vi "Test RedCase_FlashUpdate_Run.bat.vi"(8 "error in (no error)":errorcluster, 9 "SN":string="ABCSN", 10 "RedCase Auto Path":string=".\\RedCase_Auto\\Debug\\FlashUpdate_Run.bat", 11 "Bin":string=".\\RedCase_Auto\\Debug\\HX6330B03_C_Sharp_GM_Mobis_2992x1299_16.3_Falcon_20251223_S1C7A404_Test_Ver4-0.bin") -> (0 "error out":errorcluster, 2 "RecCase Log Path":string, 3 "Result":bool)   [LabVIEW 2024]
uses:
  <vilib>/Utility/error.llb/Trim Whitespace One-Sided.vi
panel:
  out "output Str":string="@echo off\nsetlocal enabledelayedexpansion\n\nREM ========= 用户可配置区 =========\nset RFP_DIR=C:\\Program Files (x86)\\Renesas Electronics\\Programming Tools\\Renesas Flash Programmer V3.16\nset RFP_EXE=%RFP_DIR%\\RFPV3.exe\nset RFP_CONSOLE=%RFP_DIR%\\RFPV3.Console.exe\n\nset PROJECT=D:\\Alvin\\1.Project\\5.ZhiRuiJia\\Flash\\RFP_Auto\\Project\\k7001.rpj\nREM 固件已配置在 .rpj 内，这里默认不再单独指定 /file\nset FIRMWARE=\nset LOG_DIR=D:\\Alvin\\1.Project\\5.ZhiRuiJia\\Flash\\RFP_Auto\\Logs\nset RETRY=2\nREM 可选：如果你只有一台E2 Lite，通常不需要指定tool序列号\nset TOOL_SN=\nREM 示例：set TOOL_SN=xxxxxxxxx\nREM =================================\n\nif not exist \"%LOG_DIR%\" mkdir \"%LOG_DIR%\"\n\nREM SN 可由扫码枪/上位机传入：flash_once.bat SNABCSN\nset SN=%1\nif \"%SN%\"==\"\" set SN=NO_SN\n\nREM 时间戳（yyyyMMdd_HHmmss）\nfor /f %%i in ('powershell -NoProfile -Command \"Get-Date -Format yyyyMMdd_HHmmss\"') do set TS=%%i\n\nset LOG_FILE=%LOG_DIR%\\%SN%_%TS%.log\n\necho [INFO] SN=%SN%\necho [INFO] Project=%PROJECT%\nif not \"%FIRMWARE%\"==\"\" echo [INFO] Firmware=%FIRMWARE%\necho [INFO] Log=%LOG_FILE%\necho.\n\nREM 参数拼接\nset COMMON_ARGS=/silent \"%PROJECT%\" /command epv /log \"%LOG_FILE%\"\nif not \"%FIRMWARE%\"==\"\" set COMMON_ARGS=%COMMON_ARGS% /file \"%FIRMWARE%\"\nif not \"%TOOL_SN%\"==\"\" set COMMON_ARGS=%COMMON_ARGS% /tool %TOOL_SN%\n\nset /a COUNT=0\n\n:RETRY_LOOP\nset /a COUNT+=1\necho [INFO] Attempt !COUNT! ...\n\nREM 优先用 RFPV3.exe /silent\n\"%RFP_EXE%\" %COMMON_ARGS%\nset RC=%ERRORLEVEL%\n\necho [INFO] ExitCode=%RC%\n\nif \"%RC%\"==\"0\" goto PASS\n\nif !COUNT! LEQ %RETRY% (\n    echo [WARN] Programming failed, retrying...\n    timeout /t 2 >nul\n    goto RETRY_LOOP\n)\n\ngoto FAIL\n\n:PASS\nfor /f %%i in ('powershell -NoProfile -Command \"Get-Date -Format yyyyMMdd_HHmmss\"') do set END_TS=%%i\necho [INFO] EndTime=%END_TS%\necho [PASS] %SN% %TS% >> \"%LOG_DIR%\\summary_pass.txt\"\necho SUCCESS\nexit /b 0\n\n:FAIL\nfor /f %%i in ('powershell -NoProfile -Command \"Get-Date -Format yyyyMMdd_HHmmss\"') do set END_TS=%%i\necho [INFO] EndTime=%END_TS%\necho [FAIL] %SN% %TS% ExitCode=%RC% >> \"%LOG_DIR%\\summary_fail.txt\"\necho FAIL\nexit /b 1\r\n"
  out "path":path=path "D:/WeiFu/Labview ATS/Customer_Zhuo/RF_Download/ATS/Project/RFP_Auto/Scripts/Flash_once.bat"
  out "result string":string
  # "D:\\WeiFu\\Labview ATS\\Customer_Zhuo\\RF_Download\\ATS\\Project\\RFP_Auto\\Scripts\\Flash_once.bat"
  # "..\\RFP_Auto\\Scripts\\Flash_once.bat"
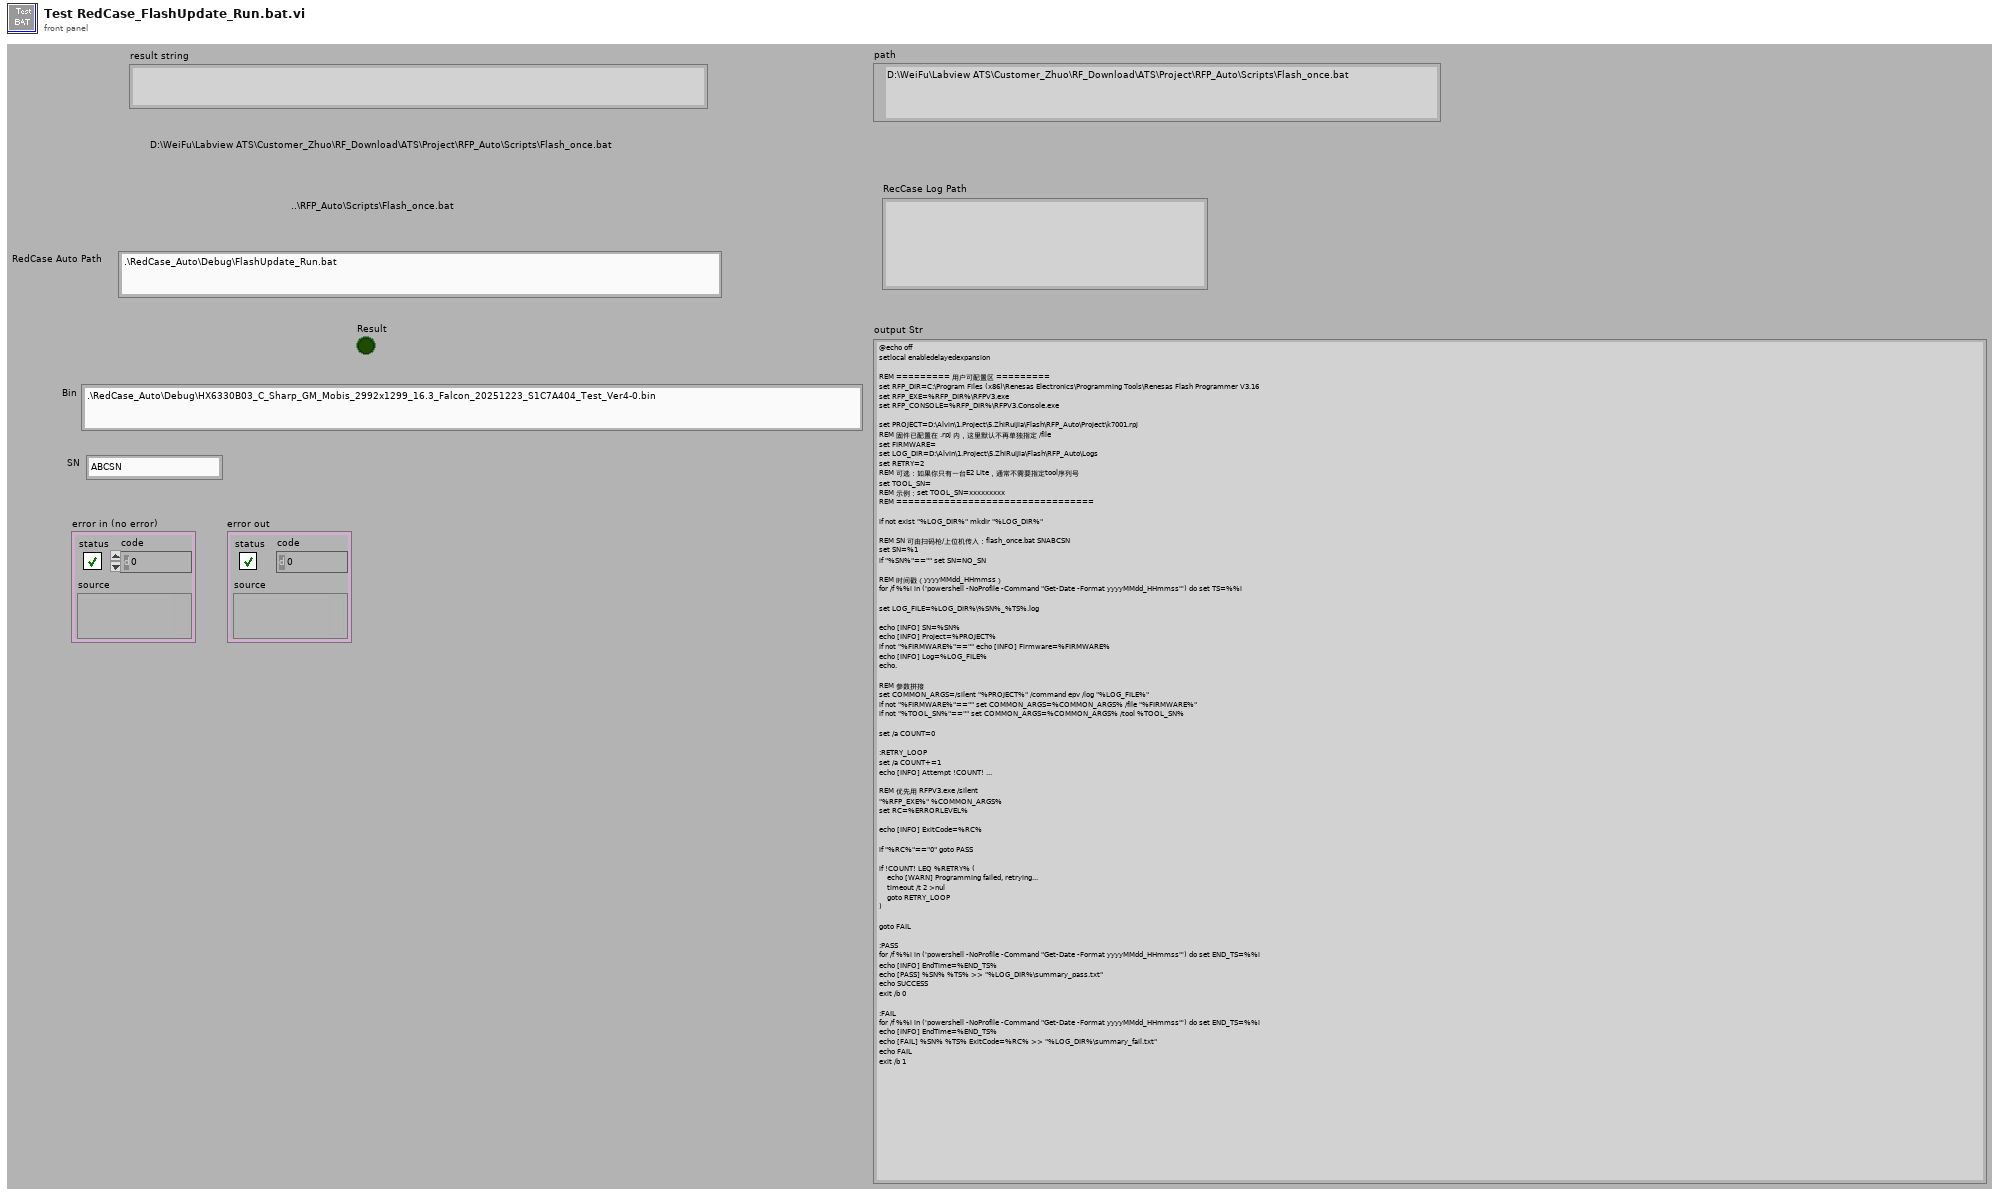
[diagram p1: front panel]
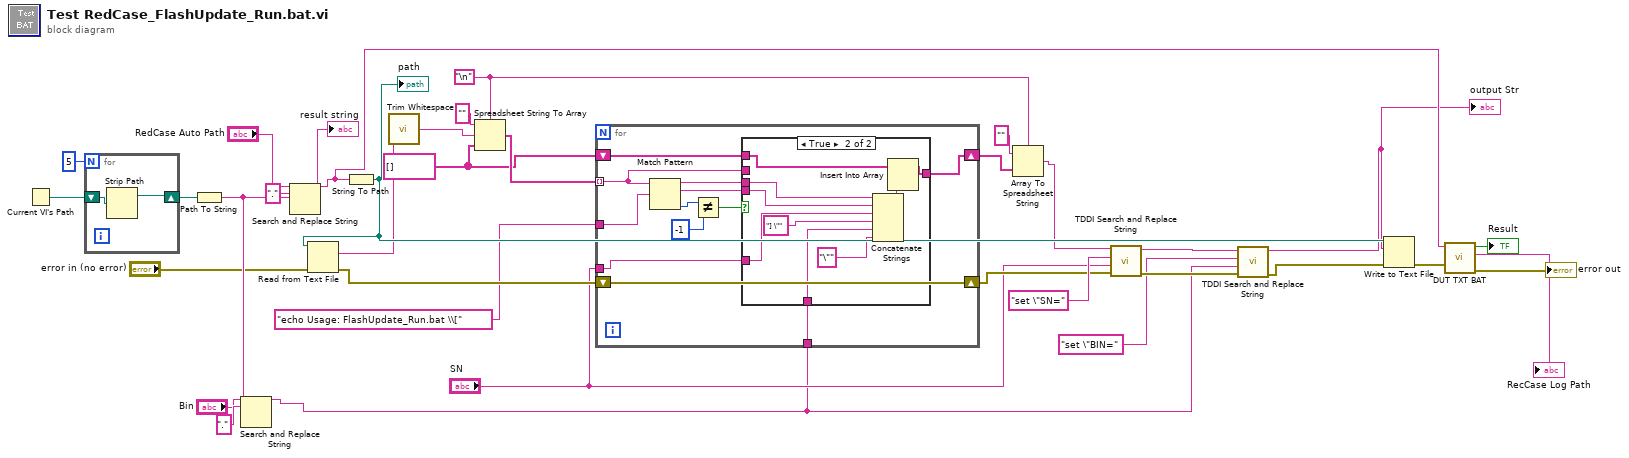
[diagram p0: block diagram]
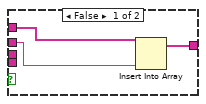
[diagram p2: hidden frame]
diagram:
  w18 = string[] []
  w15 = "\n"
  n1 = Current VI's Path() -> (path=w33:path)
  n2 = for {
    N: 5 -> [_]
    shift-right: [w36] -> w31
    shift-left: w33 -> [w37]
    n3 = Strip Path(path=w37) -> (stripped path=w36:path)  [unwired: 1 out]
  }
  n4 = Path To String(path=w31) -> (string=w26:string)
  n5 = Search and Replace String(input string="Bin", search string=".", replace string=w26) -> (result string=w1:string)  [unwired: 5 in, 3 out]
  n6 = Search and Replace String(input string="RedCase Auto Path", search string=".", replace string=w26) -> (result string=w11:string)  [unwired: 5 in, 3 out]
  "result string" <- w11
  n7 = String To Path(string=w11) -> (path=w22:path)
  "path" <- w22
  n8 = Read from Text File(file (use dialog)=w22, error in="error in (no error)") -> (text=w14:string, error out=w13:errorcluster)  [unwired: 2 in, 2 out]
  n9 = call <vilib>:"Trim Whitespace.vi"("string"=w14) -> ("trimmed string"=w20:string)  [unwired: 1 in]
  n10 = Spreadsheet String To Array(delimiter (Tab)=w15, format string="", spreadsheet string=w20, array type (2D Dbl)=w18) -> (array=w19:string[])
  n11 = for {
    tunnel: w19 -> [w46] mode=indexing
    tunnel: "echo Usage: FlashUpdate_Run.bat \\[" ("search string") -> [w49]
    shift-right: [w44] -> w17
    shift-left: w18 -> [w45]
    tunnel: "SN" -> [w40]
    shift-right: [w39] -> w9
    shift-left: w13 -> [w39]
    tunnel: w1 -> [w38]
    n12 = Match Pattern(string=w46, regular expression=w49) -> (before substring=w42:string, match substring=w41:string, offset past match=w43:i32)  [unwired: 1 in, 1 out]
    n13 = Not Equal?(x=w43, y=-1) -> (x != y?=w47:bool)
    n14 = case shown="True" w47 {
      tunnel: w46 -> [w51 _]
      tunnel: w45 -> [w52 w59]
      tunnel: [w50 w57] -> w44
      tunnel: w42 -> [_ w61]
      tunnel: w41 -> [_ w60]
      tunnel: w40 -> [_ w56]
      tunnel: w38 -> [_ w54]
      frame False {
        n15 = Insert Into Array(array=w52, new element=w51) -> (w50:string[])  [unwired: 1 in]
      }
      frame True {
        n16 = Concatenate Strings(w61, w60, w56, "] \"" ("format string"), w54, "\"" ("string")) -> (w58:string)
        n17 = Insert Into Array(array=w59, new element=w58) -> (w57:string[])  [unwired: 1 in]
      }
    }
  }
  n18 = Array To Spreadsheet String(delimiter (Tab)=w15, array=w17, 3:"" ("format string")) -> (spreadsheet string=w8:string)
  n19 = call "TDDI Search and Replace String.vi"("error in (no error)"=w9, "Replace Str"="SN", "FindStr"="set \"SN=" ("string"), "originalTex"=w8) -> ("error out"=w7:errorcluster, "output Str"=w6:string)  [unwired: 6 in]
  n20 = call "TDDI Search and Replace String.vi"("error in (no error)"=w7, "Replace Str"=w1, "FindStr"="set \"BIN=", "originalTex"=w6) -> ("error out"=w2:errorcluster, "output Str"=w5:string)  [unwired: 6 in]
  "output Str" <- w5
  n21 = Write to Text File(file (use dialog)=w22, text=w5, error in=w2) -> (error out=w24:errorcluster)  [unwired: 1 in, 2 out]
  n22 = call "DUT TXT BAT.vi"("error in (no error)"=w24, "command line"=w11) -> ("error out"=→"error out":errorcluster, "Log Path"=→"RecCase Log Path":string, "Result"=→"Result":bool)  [unwired: 7 in]
